vi "pmu_Check Trigger Limits.vi"(8 "error in (no error)":errorcluster, 10 "phasors in":csg[](array[numeric]), 11 "trigger limits in":T1={"magnitude and phase"=[], "freq. upper limit (Hz)"=70.0, "freq. lower limit (Hz)"=40.0, "rate of change limit (Hz/s)"=323.67}) -> (0 "error out":errorcluster, 2 "phasors out":csg[](array[numeric]), 3 "trigger limits out":T1={"magnitude and phase"=[], "freq. upper limit (Hz)"=70.0, "freq. lower limit (Hz)"=40.0, "rate of change limit (Hz/s)"=323.67})   [LabVIEW 2011, in "NI_EP_PMU.lvlib"]
uses:
  <vilib>/addons/Electrical Power/PMU/NI_EP_PMU.lvlib
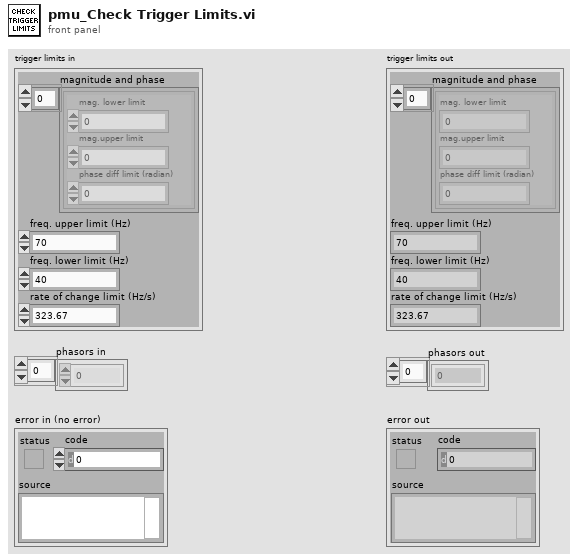
[diagram p1: front panel]
types:
  T1 = cluster{"magnitude and phase":cluster{"mag. lower limit":sgl, "mag.upper limit":sgl, "phase diff limit (radian)":sgl}[], "freq. upper limit (Hz)":sgl, "freq. lower limit (Hz)":sgl, "rate of change limit (Hz/s)":sgl}
  T2 = cluster{"mag. lower limit":sgl, "mag.upper limit":sgl, "phase diff limit (radian)":sgl}[]
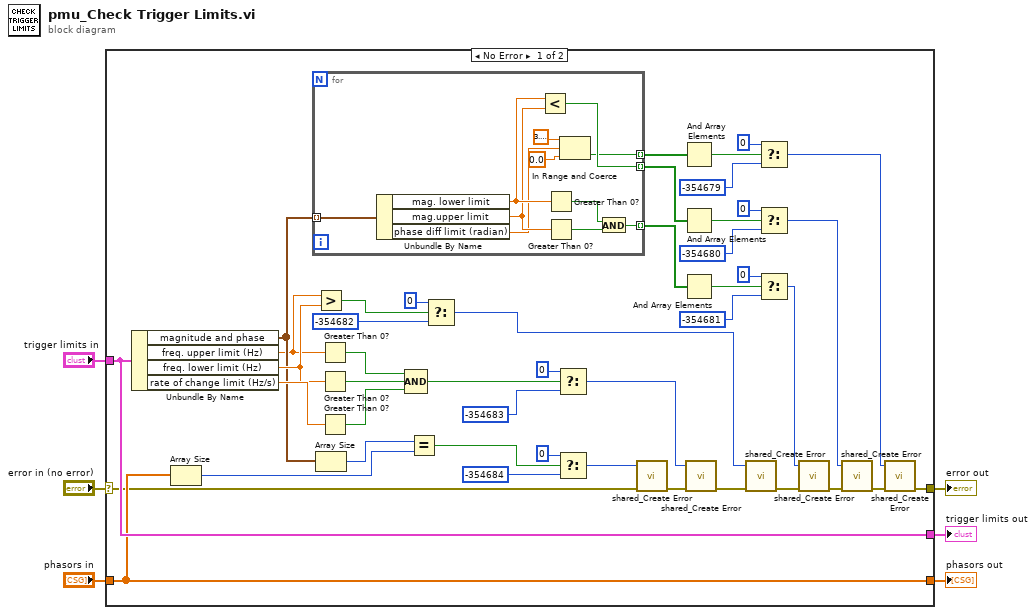
[diagram p0: block diagram]
diagram:
  n1 = case shown="No Error" "error in (no error)" {
    selector: "error in (no error)" -> [w23 w65]
    tunnel: "trigger limits in" -> [w34 w63]
    tunnel: "phasors in" -> [w32 w64]
    tunnel: [w7 w65] -> w3
    tunnel: [w32 w64] -> w2
    tunnel: [w34 w63] -> w1
    frame No Error {
      n2 = Unbundle By Name(w34) -> ("magnitude and phase"=w41:T2, "freq. upper limit (Hz)"=w33:sgl, "freq. lower limit (Hz)"=w43:sgl, "rate of change limit (Hz/s)"=w45:sgl)
      n3 = Array Size(array=w32) -> (size(s)=w51:i32)
      n4 = for {
        tunnel: w41 -> [w62] mode=indexing
        tunnel: [w59] -> w37 mode=indexing
        tunnel: [w58] -> w39 mode=indexing
        tunnel: [w52] -> w36 mode=indexing
        n5 = Unbundle By Name(w62) -> ("mag. lower limit"=w57:sgl, "mag.upper limit"=w56:sgl, "phase diff limit (radian)"=w55:sgl)
        n6 = Less?(x=w57, y=w56) -> (x < y?=w58:bool)
        n7 = Greater Than 0?(x=w57) -> (x > 0?=w61:bool)
        n8 = Greater Than 0?(x=w56) -> (x > 0?=w60:bool)
        n9 = In Range and Coerce(upper limit=sgl 3.1415927, x=w55, lower limit=sgl 0.0 ("upper limit")) -> (In Range?=w52:bool)  [unwired: 1 out]
        n10 = And(x=w61, y=w60) -> (x .and. y?=w59:bool)
      }
      n11 = Greater?(x=w33, y=w43) -> (0:w42:bool)
      n12 = Array Size(array=w41) -> (size(s)=w50:i32)
      n13 = Greater Than 0?(x=w33) -> (x > 0?=w48:bool)
      n14 = Greater Than 0?(x=w43) -> (x > 0?=w47:bool)
      n15 = Greater Than 0?(x=w45) -> (x > 0?=w44:bool)
      n16 = Compound Arithmetic op=AND(w48, w47, w44) -> (w46:bool)
      n17 = Equal?(x=w50, y=w51) -> (x = y?=w49:bool)
      n18 = Select(t=0 ("error code (0)"), s=w42, f=-354682 ("error code (0)")) -> (s? t:f=w18:i32)
      n19 = Select(t=0 ("error code (0)"), s=w46, f=-354683 ("error code (0)")) -> (s? t:f=w22:i32)
      n20 = Select(t=0 ("error code (0)"), s=w49, f=-354684 ("error code (0)")) -> (s? t:f=w24:i32)
      n21 = call <vilib>:"shared_Create Error.vi"("error in (no error)"=w23, "error code (0)"=w24) -> ("error out"=w20:errorcluster)  [unwired: 9 in]
      n22 = And Array Elements(Boolean array=w36) -> (logical AND=w35:bool)
      n23 = And Array Elements(Boolean array=w39) -> (logical AND=w38:bool)
      n24 = And Array Elements(Boolean array=w37) -> (logical AND=w40:bool)
      n25 = call <vilib>:"shared_Create Error.vi"("error in (no error)"=w20, "error code (0)"=w22) -> ("error out"=w17:errorcluster)  [unwired: 9 in]
      n26 = call <vilib>:"shared_Create Error.vi"("error in (no error)"=w17, "error code (0)"=w18) -> ("error out"=w15:errorcluster)  [unwired: 9 in]
      n27 = Select(t=0 ("error code (0)"), s=w35, f=-354679 ("error code (0)")) -> (s? t:f=w8:i32)
      n28 = Select(t=0 ("error code (0)"), s=w38, f=-354680 ("error code (0)")) -> (s? t:f=w11:i32)
      n29 = Select(t=0 ("error code (0)"), s=w40, f=-354681 ("error code (0)")) -> (s? t:f=w14:i32)
      n30 = call <vilib>:"shared_Create Error.vi"("error in (no error)"=w15, "error code (0)"=w14) -> ("error out"=w12:errorcluster)  [unwired: 9 in]
      n31 = call <vilib>:"shared_Create Error.vi"("error in (no error)"=w12, "error code (0)"=w11) -> ("error out"=w9:errorcluster)  [unwired: 9 in]
      n32 = call <vilib>:"shared_Create Error.vi"("error in (no error)"=w9, "error code (0)"=w8) -> ("error out"=w7:errorcluster)  [unwired: 9 in]
    }
    frame Error {
    }
  }
  "error out" <- w3
  "trigger limits out" <- w1
  "phasors out" <- w2
